vi "wait.vi"(9 "Input \nparameters":T3={"Frame rate (ms)"=2000, "Worm strain"="N2", "Time t"=0, "State"=enum."Image acquisition", "Acquisition time"=0.0, "Max_num_runs"=100000, "#TTL"=0, "Time of start TTL"=100000, "ImSub Value"=0, "Time of last TTL"=0, "Number of Columns"=2, "Number of Rows"=2, "# AdjacentTTL"=0, "Sleep deprivation status"="", "Sleep Detection"=FALSE, "# Sleep detections"=0, "Time of first sleep detection"=0, "Time max # adjacent TTL"=0, "Image t-1"=[], "Image t"=[]} {"Number of Rows" items=["1"=1, "2"=2, "3"=3, "4"=4]; "Number of Columns" items=["1"=1, "2"=2, "3"=3, "4"=4]}) -> (1 "Output \nparameters":T2={"Frame rate (ms)"=2000, "Worm strain"="N2", "Time t"=0, "State"=enum."Image acquisition", "Time elapsed"=0.0, "Max_num_runs"=100000, "#TTL"=0, "Time of start TTL"=100000, "ImSub Value"=0, "Time of last TTL"=0, "Number of Columns"=2, "Number of Rows"=2, "# AdjacentTTL"=0, "Sleep deprivation status"="", "Sleep Detection"=FALSE, "# Sleep detections"=0, "Time of first sleep detection"=0, "Time max # adjacent TTL"=0, "Image t-1"=[], "Image t"=[]} {"Number of Rows" items=["1"=1, "2"=2, "3"=3, "4"=4]; "Number of Columns" items=["1"=1, "2"=2, "3"=3, "4"=4]}, 3 "Wait":bool)   [LabVIEW 2011]
uses:
  state.ctl
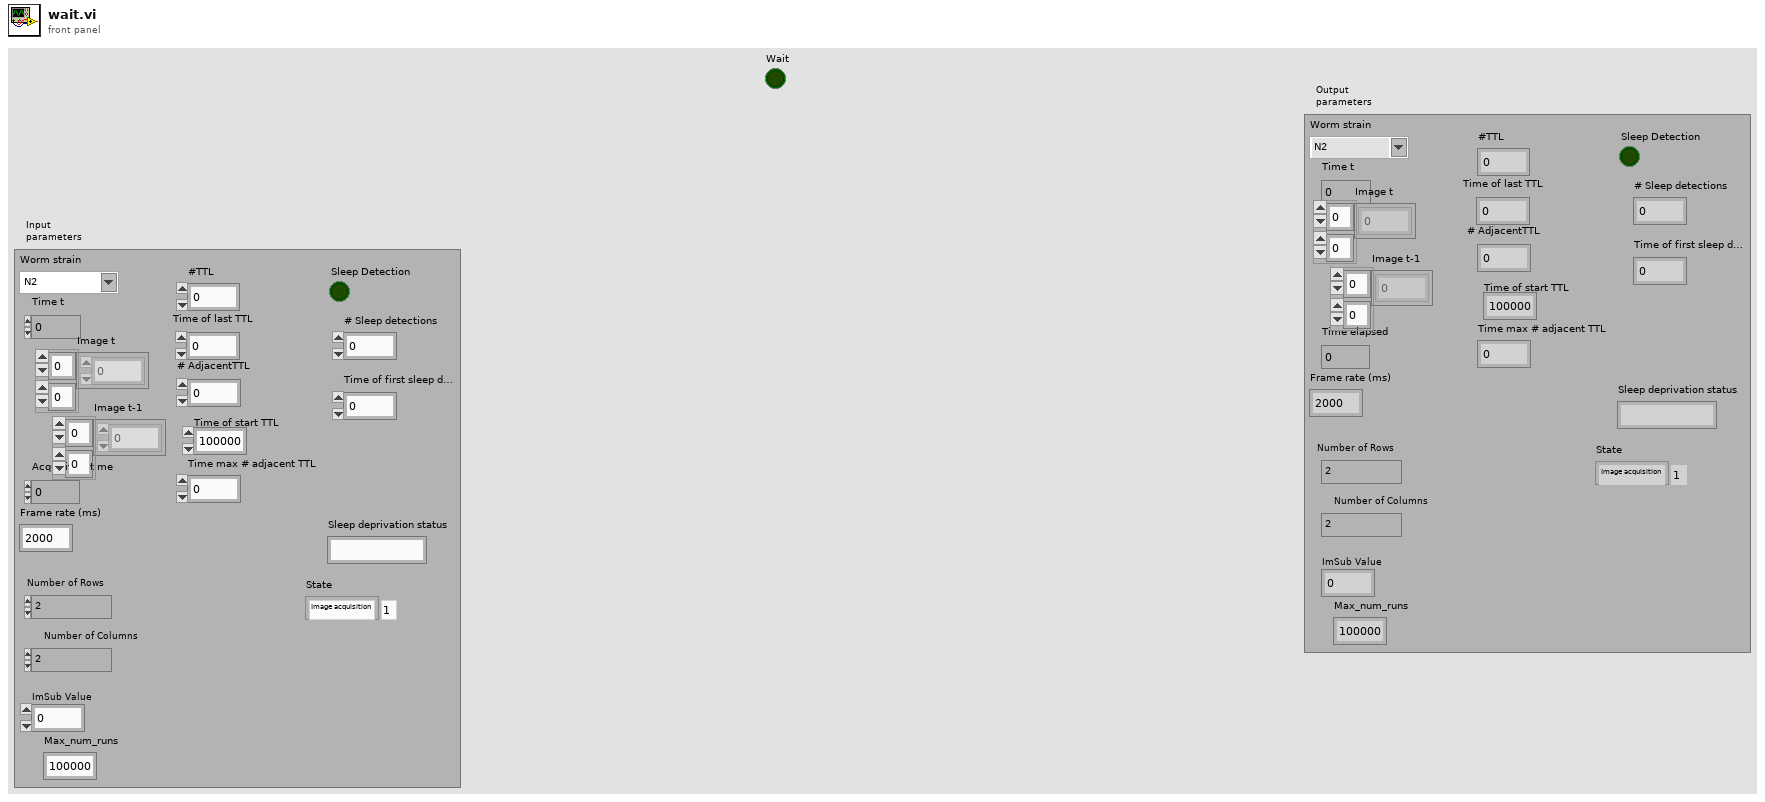
[diagram p1: front panel]
types:
  T1 = typedef "state.ctl" = enum16{"Initialize measurement", "Image acquisition", "Image processing", "Sleep detection", "Control TTL protocol ", "Sleep deprivation", "Update image & exit condition", "Wait "}
  T2 = cluster{"Frame rate (ms)":u32, "Worm strain":string, "Time t":i32, "State":T1, "Time elapsed":dbl, "Max_num_runs":i32, "#TTL":i32, "Time of start TTL":i32, "ImSub Value":i32, "Time of last TTL":i32, "Number of Columns":u32, "Number of Rows":u32, "# AdjacentTTL":i32, "Sleep deprivation status":string, "Sleep Detection":bool, "# Sleep detections":i32, "Time of first sleep detection":i32, "Time max # adjacent TTL":i32, "Image t-1":i32[][], "Image t":i32[][]}
  T3 = cluster{"Frame rate (ms)":u32, "Worm strain":string, "Time t":i32, "State":T1, "Acquisition time":dbl, "Max_num_runs":i32, "#TTL":i32, "Time of start TTL":i32, "ImSub Value":i32, "Time of last TTL":i32, "Number of Columns":u32, "Number of Rows":u32, "# AdjacentTTL":i32, "Sleep deprivation status":string, "Sleep Detection":bool, "# Sleep detections":i32, "Time of first sleep detection":i32, "Time max # adjacent TTL":i32, "Image t-1":i32[][], "Image t":i32[][]}
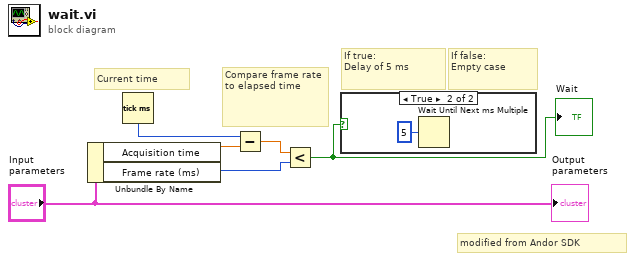
[diagram p0: block diagram]
diagram:
  # "modified from Andor SDK"
  # "Current time"
  # "If false: \nEmpty case"
  # "If true: \nDelay of 5 ms"
  # "Compare frame rate to elapsed time"
  n1 = Unbundle By Name("Input \nparameters") -> ("Acquisition time"=w4:dbl, "Frame rate (ms)"=w6:u32)
  n2 = Tick Count (ms) ("Initial Tick Count (ms)")() -> (millisecond timer value=w5:u32)
  n3 = Subtract(x=w5, y=w4) -> (x-y=w3:dbl)
  n4 = Less?(x=w3, y=w6) -> (x < y?=w2:bool)
  "Wait" <- w2
  n5 = case shown="True" w2 {
    frame False {
    }
    frame True {
      n6 = Wait Until Next ms Multiple(millisecond multiple=u32 5 ("Vielfache von ms")) -> ()  [unwired: 1 out]
    }
  }
  "Output \nparameters" <- "Input \nparameters"
